vi "DSO1K Acquire Multiple Waveforms.vi"() -> ()   [LabVIEW 2009]
doc: "This example shows how to configure multiple channels and acquire waveforms from multiple channels."
uses:
  <instrlib>/DSO1K/DSO1K.lvlib
panel:
  in  "Timeout (40000 ms)":u32=40000
  in  "Timebase (12:10us)":u16(ring)=12 items=["1ns", "2ns", "5ns", "10ns", "20ns", "50ns", "100ns", "200ns", "500ns", "1us", "2us", "5us", "10us", "20us", "50us", "100us", "200us", "500us", "1ms", "2ms", "5ms", "10ms", "20ms", "50ms", "100ms", "200ms", "500ms", "1s", "2s", "5s", "10s", "20s", "50s", "100s"]
  in  "Probe Attenuation (9:1X)":u16(ring)=9 items=["0.001 X", "0.002 X", "0.005 X", "0.01 X", "0.02 X", "0.05 X", "0.1 X", "0.2 X", "0.5 X", "1 X", "2 X", "5 X", "10 X", "20 X", "50 X", "100 X", "200 X", "500 X", "1k X"]
  in  "Vertical Coupling (0: DC)":u16(ring) items=["DC", "AC", "Ground"]
  in  "Vertical Range (100m)":dbl=0.1 format="%#_4p"
  in  "Channel (1: Channel 2)":u16(ring)=2 items=["Channel 1"=1, "Channel 2"=2, "Channel 3"=3, "Channel 4"=4]
  in  "Probe Attenuation (9:1X)":u16(ring)=9 items=["0.001 X", "0.002 X", "0.005 X", "0.01 X", "0.02 X", "0.05 X", "0.1 X", "0.2 X", "0.5 X", "1 X", "2 X", "5 X", "10 X", "20 X", "50 X", "100 X", "200 X", "500 X", "1k X"]
  in  "Vertical Coupling (0: DC)":u16(ring) items=["DC", "AC", "Ground"]
  in  "Vertical Range (100m)":dbl=0.1 format="%#_4p"
  in  "Channel (1: Channel 1)":u16(ring)=1 items=["Channel 1"=1, "Channel 2"=2, "Channel 3"=3, "Channel 4"=4]
  out "Waveform Graph":cluster{dbl, "Sampling Period":dbl, dbl[]}[](graph)
  in  "VISA resource name":refnum<visa-resource-name>
  # "Channel A"
  # "Channel B"
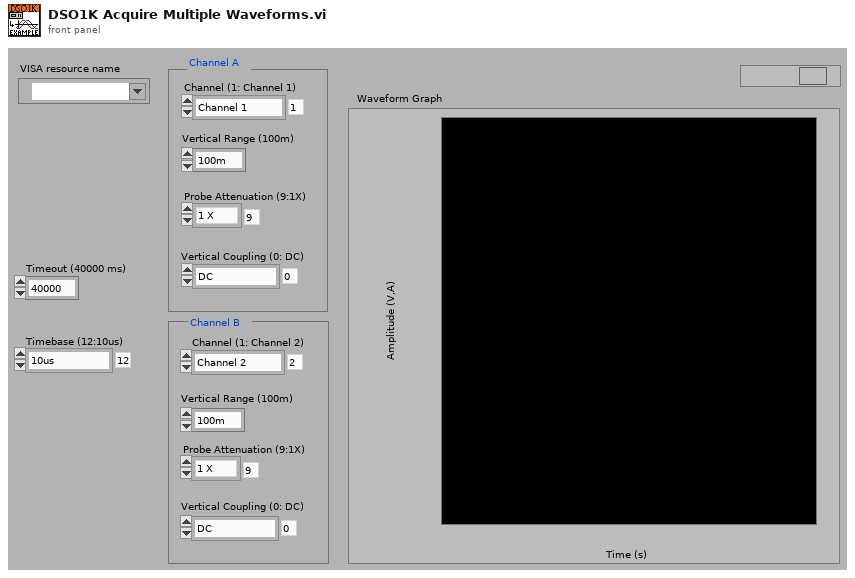
[diagram p1: front panel]
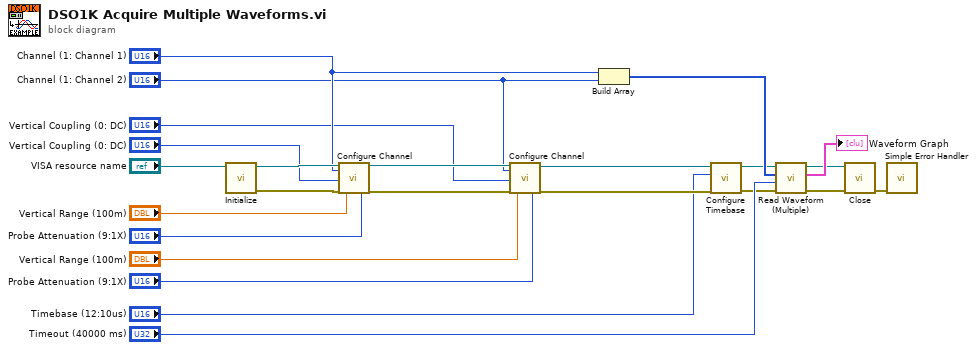
[diagram p0: block diagram]
diagram:
  n1 = call <instrlib>:"Initialize.vi"("VISA resource name"="VISA resource name") -> ("error out"=w20:errorcluster, "VISA resource name out"=w19:refnum<visa-resource-name>)  [unwired: 9 in]
  n2 = call <instrlib>:"Configure Channel.vi"("VISA resource name"=w19, "Channel (1: Channel 1)"="Channel (1: Channel 1)", "Vertical Coupling (0: DC)"="Vertical Coupling (0: DC)", "error in (no error)"=w20, "Vertical Range (100m)"="Vertical Range (100m)", "Probe Attenuation (9:1X)"="Probe Attenuation (9:1X)") -> ("VISA resource name out"=w18:refnum<visa-resource-name>, "error out"=w17:errorcluster)  [unwired: 12 in]
  n3 = call <instrlib>:"Configure Channel.vi"("VISA resource name"=w18, "Channel (1: Channel 1)"="Channel (1: Channel 2)", "Vertical Coupling (0: DC)"="Vertical Coupling (0: DC)", "error in (no error)"=w17, "Vertical Range (100m)"="Vertical Range (100m)", "Probe Attenuation (9:1X)"="Probe Attenuation (9:1X)") -> ("VISA resource name out"=w22:refnum<visa-resource-name>, "error out"=w21:errorcluster)  [unwired: 12 in]
  n4 = Build Array("Channel (1: Channel 1)", "Channel (1: Channel 2)") -> (w7:u16[])
  n5 = call <instrlib>:"Configure Timebase.vi"("error in (no error)"=w21, "Timebase (12:10us)"="Timebase (12:10us)", "VISA resource name"=w22) -> ("error out"=w4:errorcluster, "VISA resource name out"=w5:refnum<visa-resource-name>)  [unwired: 7 in]
  n6 = call <instrlib>:"Read Waveform (Multiple).vi"("error in (no error)"=w4, "Timeout (40000 ms)"="Timeout (40000 ms)", "Channels"=w7, "VISA resource name"=w5) -> ("error out"=w3:errorcluster, "Waveform Graph"=→"Waveform Graph":cluster{dbl, "Sampling Period":dbl, dbl[]}[], "VISA resource name out"=w1:refnum<visa-resource-name>)  [unwired: 4 in, 1 out]
  n7 = call <instrlib>:"Close.vi"("error in (no error)"=w3, "VISA resource name"=w1) -> ("error out"=w23:errorcluster)  [unwired: 9 in]
  n8 = call <vilib>:"Simple Error Handler.vi"("error in (no error)"=w23) -> ()  [unwired: 4 in, 5 out]
